vi "初始化Global.vi"(8 "error in (no error)":errorcluster) -> (0 "error out":errorcluster)   [LabVIEW 2015]
uses:
  Global/SeverGlobal.vi
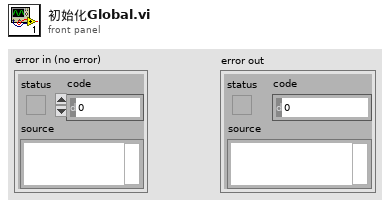
[diagram p1: front panel]
types:
  T1 = cluster{"TCP Ref":refnum<k5>, "Broadcast":refnum<k5>, "Broadcast 2":refnum<k5>, "IP":string, "port":u16, "userName":string, "passWord":string, "authority":string}[]
  T2 = cluster{"TCP Ref":refnum<k5>, "IP":string, "userName":string, "IN":u16, "OUT":u16, "time":u32}[]
  T3 = cluster{"TCP Ref":refnum<k5>, "IP":string, "userName":string, "A":u16, "COM":u16, "time":u32}[]
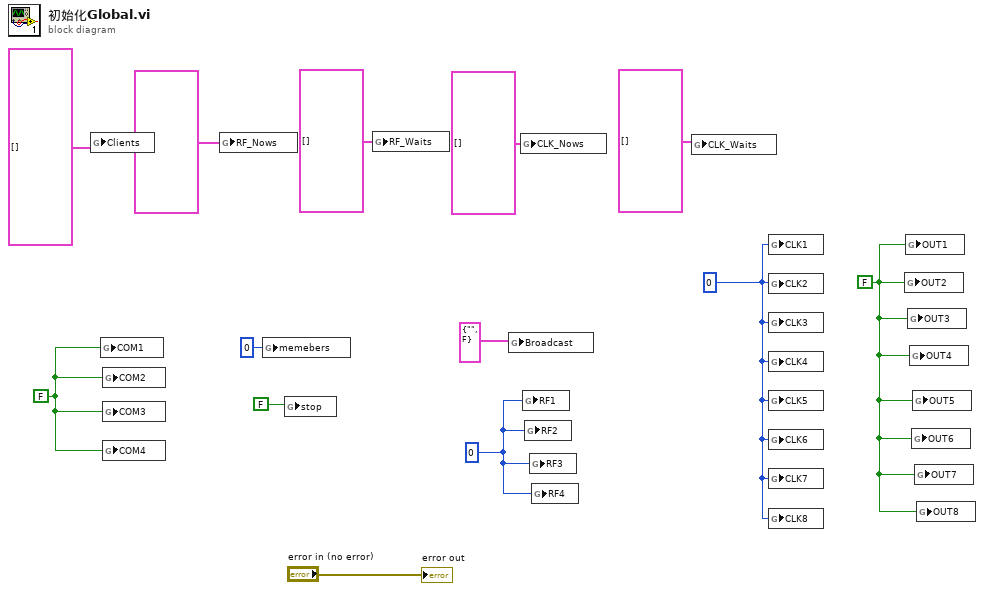
[diagram p0: block diagram]
diagram:
  w1 = FALSE
  w2 = 0 ("memebers")
  w3 = 0 ("memebers")
  w7 = FALSE
  n1 = global write "SeverGlobal.vi" "Clients"(T1 [] ("Clients")) -> ()
  n2 = global write "SeverGlobal.vi" "COM1"(w7) -> ()
  n3 = global write "SeverGlobal.vi" "COM2"(w7) -> ()
  n4 = global write "SeverGlobal.vi" "COM3"(w7) -> ()
  n5 = global write "SeverGlobal.vi" "COM4"(w7) -> ()
  n6 = global write "SeverGlobal.vi" "RF_Nows"(T3 [] ("RF_Nows")) -> ()
  n7 = global write "SeverGlobal.vi" "memebers"(0 ("memebers")) -> ()
  n8 = global write "SeverGlobal.vi" "stop"(FALSE ("stop")) -> ()
  n9 = global write "SeverGlobal.vi" "RF_Waits"(T3 [] ("RF_Waits")) -> ()
  n10 = global write "SeverGlobal.vi" "Broadcast"(cluster{"消息类型":string, "广播？":bool} {"消息类型"="", "广播？"=FALSE} ("Broadcast")) -> ()
  n11 = global write "SeverGlobal.vi" "CLK_Nows"(T2 [] ("CLK_Nows")) -> ()
  n12 = global write "SeverGlobal.vi" "RF1"(w3) -> ()
  n13 = global write "SeverGlobal.vi" "RF2"(w3) -> ()
  n14 = global write "SeverGlobal.vi" "RF3"(w3) -> ()
  n15 = global write "SeverGlobal.vi" "RF4"(w3) -> ()
  n16 = global write "SeverGlobal.vi" "CLK_Waits"(T2 [] ("CLK_Waits")) -> ()
  n17 = global write "SeverGlobal.vi" "CLK1"(w2) -> ()
  n18 = global write "SeverGlobal.vi" "CLK2"(w2) -> ()
  n19 = global write "SeverGlobal.vi" "CLK3"(w2) -> ()
  n20 = global write "SeverGlobal.vi" "CLK4"(w2) -> ()
  n21 = global write "SeverGlobal.vi" "CLK5"(w2) -> ()
  n22 = global write "SeverGlobal.vi" "CLK6"(w2) -> ()
  n23 = global write "SeverGlobal.vi" "CLK7"(w2) -> ()
  n24 = global write "SeverGlobal.vi" "CLK8"(w2) -> ()
  n25 = global write "SeverGlobal.vi" "OUT2"(w1) -> ()
  n26 = global write "SeverGlobal.vi" "OUT1"(w1) -> ()
  n27 = global write "SeverGlobal.vi" "OUT3"(w1) -> ()
  n28 = global write "SeverGlobal.vi" "OUT4"(w1) -> ()
  n29 = global write "SeverGlobal.vi" "OUT6"(w1) -> ()
  n30 = global write "SeverGlobal.vi" "OUT5"(w1) -> ()
  n31 = global write "SeverGlobal.vi" "OUT7"(w1) -> ()
  n32 = global write "SeverGlobal.vi" "OUT8"(w1) -> ()
  "error out" <- "error in (no error)"
